vi "Get Single Assert Display Enqueuer Reference.vi"(8 "error in (no error)":errorcluster, 10 "Assert UID":string, 11 "Main Display in":refnum<class "Main Display.lvclass">) -> (0 "error out":errorcluster, 1 "Assert Display Active?":bool, 2 "Single Assert Display Enqueuer":refnum<class "Message Enqueuer.lvclass">)   [LabVIEW 2016, in "Assert API Components.lvlib" / "Assert Display.lvlib" / "Main Display.lvlib" / "Main Display.lvclass"]
uses:
  Main Display.lvclass
  <vilib>/ActorFramework/Message Enqueuer/Message Enqueuer.lvclass
  Main Display.lvclass/Main Display.ctl
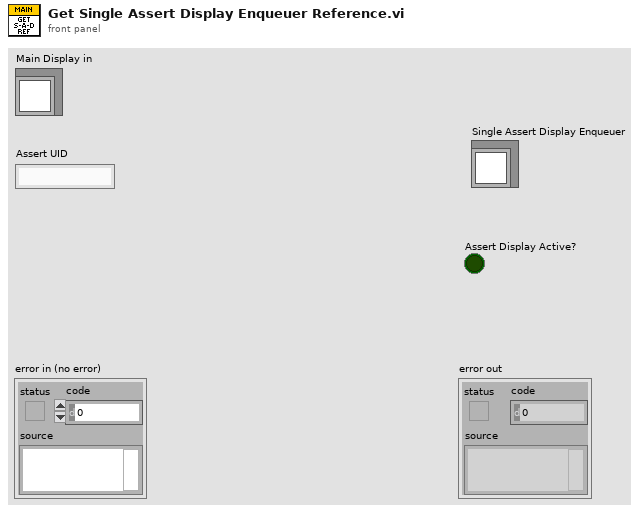
[diagram p1: front panel]
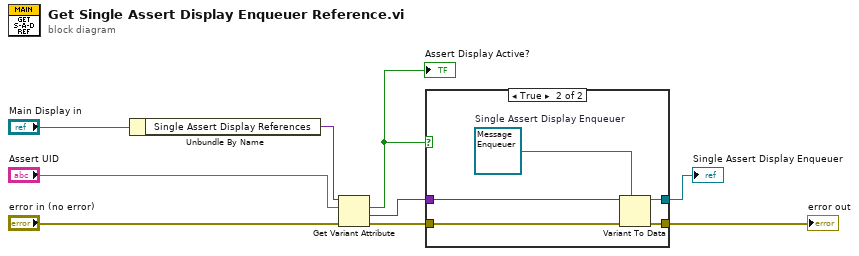
[diagram p0: block diagram]
diagram:
  n1 = Unbundle By Name("Main Display in") -> ("Single Assert Display References"=w6:variant)
  n2 = Get Variant Attribute(Variant=w6, name="Assert UID", error in="error in (no error)") -> (found=w3:bool, value=w2:variant, error out=w7:errorcluster)  [unwired: 1 in, 1 out]
  "Assert Display Active?" <- w3
  n3 = case shown="True" w3 {
    tunnel: w7 -> [w10 w15]
    tunnel: [w10 w14] -> w4
    tunnel: w2 -> [_ w13]
    tunnel: [_ w11] -> w1
    frame False {
    }
    frame True {
      w12 = refnum<class "Message Enqueuer.lvclass"> refnum  # Single Assert Display Enqueuer
      n4 = Variant To Data(error in=w15, type=w12, Variant=w13) -> (data=w11:refnum<class "Message Enqueuer.lvclass">, error out=w14:errorcluster)
    }
  }
  "error out" <- w4
  "Single Assert Display Enqueuer" <- w1
